vi "test_from_photonvision.vi"() -> ()   [LabVIEW 2020]
uses:
  PhotonVisionLib/TypeDef/PhotonPipelineResultType.ctl
  PhotonVisionLib/TypeDef/PhotonTrackedTargetType.ctl
  PhotonVisionLib/TypeDef/TargetCornerType.ctl
  <vilib>/Rock Robotics/WPI/ThirdParty/JAS_Junk/TrajLib/TypeDef/TRANSFORM2D.ctl
  <vilib>/Rock Robotics/WPI/ThirdParty/JAS_Junk/TrajLib/TypeDef/TRANSLATION2D.ctl
  <vilib>/Rock Robotics/WPI/ThirdParty/JAS_Junk/TrajLib/TypeDef/ROTATION2D.ctl
  PhotonVisionLib/PhotonVisionLib.lvlib
  <vilib>/Rock Robotics/WPI/ThirdParty/JAS_Junk/TrajLib/Trajectory_Library.lvlib
panel:
  out "PipelineResult":T1 {"Targets"."CameraToTarget"."ROTATION"."SIN" format="%13.4f"; "Targets"."CameraToTarget"."ROTATION"."COS" format="%13.4f"; "Targets"."CameraToTarget"."ROTATION"."VALUE" format="%13.4f"; "Targets"."CameraToTarget"."TRANSLATION"."Y" format="%14.3f"; "Targets"."CameraToTarget"."TRANSLATION"."X" format="%14.3f"}
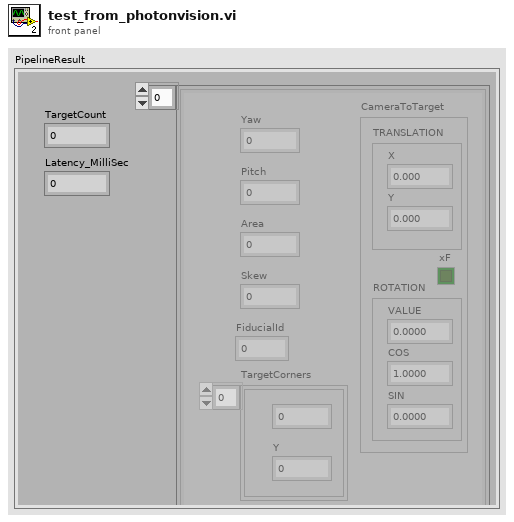
[diagram p1: front panel]
types:
  T1 = typedef "PhotonVisionLib.lvlib/PhotonPipelineResultType.ctl" = cluster{"TargetCount":i32, "Latency_MilliSec":dbl, "Targets":T2[]}
  T2 = typedef "PhotonVisionLib.lvlib/PhotonTrackedTargetType.ctl" = cluster{"Yaw":dbl, "Pitch":dbl, "Area":dbl, "Skew":dbl, "TargetCorners":T3[], "CameraToTarget":T4, "FiducialId":i32}
  T3 = typedef "PhotonVisionLib.lvlib/TargetCornerType.ctl" = cluster{"X":dbl, "Y":dbl}
  T4 = typedef "Trajectory_Library.lvlib/TRANSFORM2D.ctl" = cluster{"TRANSLATION":T5, "ROTATION":T6, "xF":bool}
  T5 = typedef "Trajectory_Library.lvlib/TRANSLATION2D.ctl" = cluster{"X":dbl, "Y":dbl}
  T6 = typedef "Trajectory_Library.lvlib/ROTATION2D.ctl" = cluster{"VALUE":dbl, "COS":dbl, "SIN":dbl}
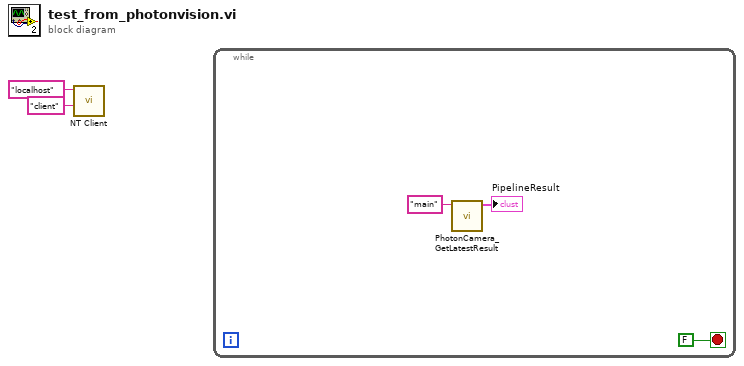
[diagram p0: block diagram]
diagram:
  n1 = call <vilib>:"NT Client.vi"("Client Name"="client", "Server IP Address"="localhost") -> ()  [unwired: 10 in]
  n2 = while {
    stop <- FALSE stop-if-true
    n3 = call "PhotonCamera_GetLatestResult.vi"("CameraName"="main") -> ("PipelineResult"=→"PipelineResult":T1)  [unwired: 9 in, 1 out]
  }
